vi "Pack5_UNDT.vi"(0 "data in":string="V4\u0012xV4\u0012\u0002\u0000\u0000\u0000pМC\u0016њwѕa\u0000\u0010\u0000‹\u0000\u0000\u0000\u0000\u0000\u0000\u0000\u0000\u0000\u0000\u0000\u0000\u0000\u0000\u0000\u0000\u0000\u0000\u0000\u0000o\u0012ѓ9\u0000\u0000\u0000\u0000\u0000\u0001\u0000\u0001+\u0019\u0000\u0001яя\"\"яяяяяяяяяяяяяяяяяяяяяяяяяяяяяяяяяяяяяяяяяяяяяяяяяяяяяяяяяяяяxV4\u0012\u0001\u0000\u0000\u0000pМC\u0016њwѕa\u0000\u0010\u0000‹\u0000\u0000\u0000\u0000\u0000\u0000\u0000\u0000\u0000\u0000\u0000\u0000\u0000\u0000\u0000\u0000\u0000\u0000\u0000\u0000o\u0012ѓ9\u0000\u0000\u0000\u0000\u0000\u0001\u0000\u0001+\u0019\u0000\u0001яя\"\u0011яяяяяяяяяяяяяяяяяяяяяяяяяяяяяяяяяяяяяяяяяяяяяяяяяяяяяяяяяяя", 5 "N tick":u8 format="%02x", 9 "OptionPACK5":T4={"MagicWordStr"="xV4\u0012", "Header size"=56, "Проверка CRC8"=TRUE, "Проверка конца пакета"=TRUE, "GainCompens"=FALSE, "Неотбрасывать BadEnd пакеты"=FALSE, "Неотбрасывать BadCRC пакеты"=FALSE, "Привести к 1"=FALSE, "GainCoef"=FALSE, "K_scale"=1.0, "ScaleOrdinate"=enum."Проценты"}, 11 "error in":errorcluster) -> (4 "data out":string, 6 "output cluster 2":T2 {"UNDT_Cluster"."Gain Coeff" format="%#_6e"; "UNDT_Cluster"."Reserve 1" format="%02x"; "UNDT_Cluster"."Mux TX/RX" format="%02x"; "UNDT_Cluster"."ScanDelay" format="%02x"; "UNDT_Cluster"."SamplingInterval" format="%#_6e"; "UNDT_Cluster"."Lose Packet" format="%08x"; "UNDT_Cluster"."EncodersParam2" format="%016x"; "UNDT_Cluster"."EncodersParam1" format="%016x"; "UNDT_Cluster"."CRC 8" format="%02x"; "UNDT_Cluster"."N chanel" format="%02x"; "UNDT_Cluster"."N tick" format="%02x"; "UNDT_Cluster"."Ncycle" format="%04x"; "UNDT_Cluster"."FrameFormatVersion" format="%02x"; "UNDT_Cluster"."MagicWord" format="%.0x"}, 8 "Status":T1={"CRC8Good"=TRUE, "PackEndGood"=TRUE, "MWFind"=TRUE, "PackToSmall"=FALSE, "offset"=4}, 10 "PackToSmall":bool, 15 "error out":errorcluster)   [LabVIEW 2017]
uses:
  Control_EU/OptionPACK5.ctl
  Control_EU/DataCluster.ctl
  Control_EU/UNDT_ClusterPackRevers (Type).ctl
  Control_EU/Status_pack5.ctl
panel:
  out "offset":i32=4
  out "SizeToSmall":bool
  out "OfsetEndPack":u32
  out "MWFind":bool=TRUE
  out "PackEndGood":bool=TRUE
  out "CRC8Good":bool=TRUE
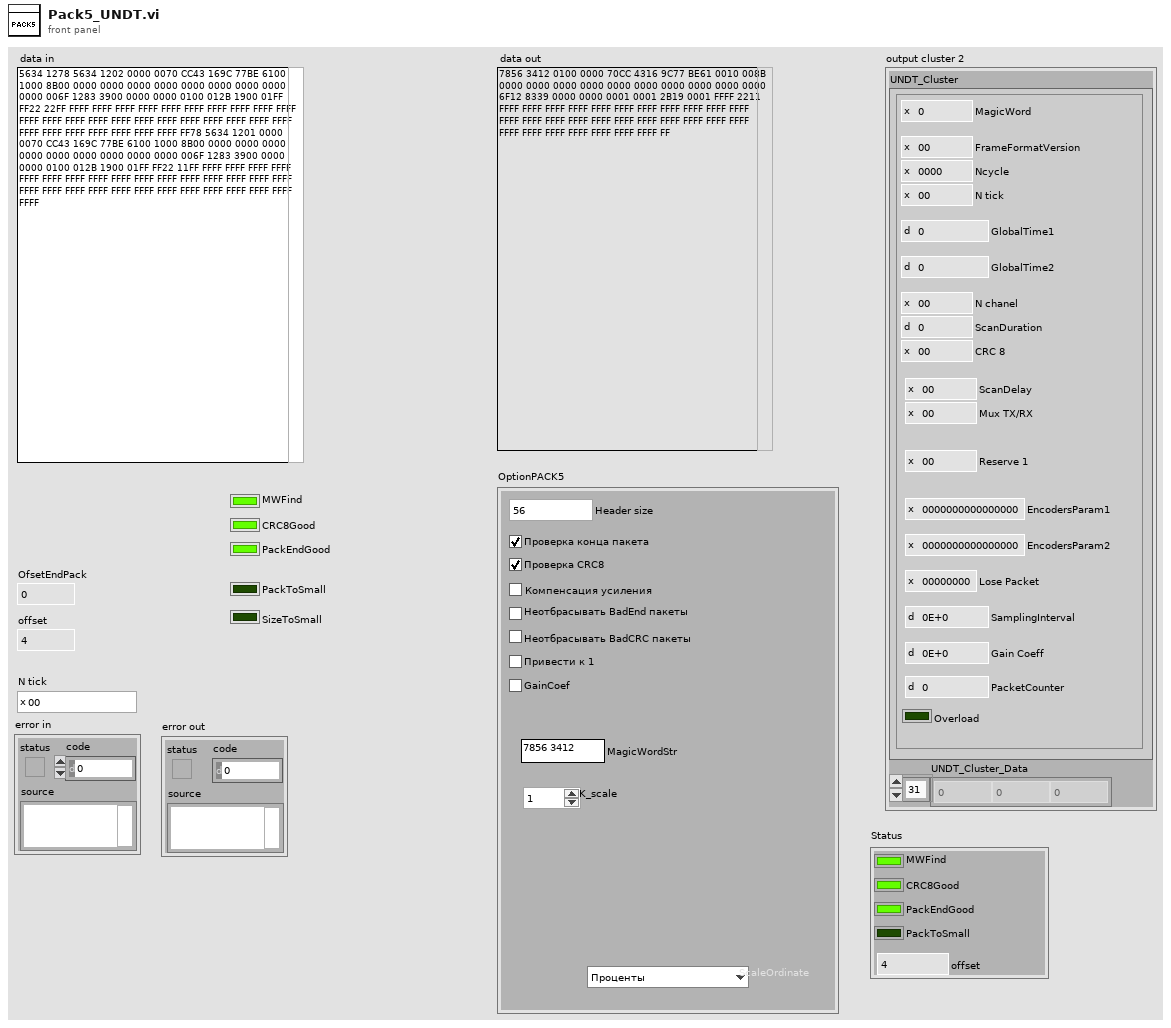
[diagram p1: front panel]
types:
  T1 = typedef "Status_pack5.ctl" = cluster{"CRC8Good":bool, "PackEndGood":bool, "MWFind":bool, "PackToSmall":bool, "offset":i32}
  T2 = typedef "DataCluster.ctl" = cluster{"UNDT_Cluster":T3, "UNDT_Cluster_Data":dbl[]}
  T3 = typedef "UNDT_ClusterPackRevers (Type).ctl" = cluster{"PacketCounter":u32, "Gain Coeff":sgl, "SamplingInterval":sgl, "Lose Packet":u32, "EncodersParam2":u64, "EncodersParam1":u64, "Reserve 1":u8, "Mux TX/RX":u8, "ScanDelay":u16, "CRC 8":u8, "ScanDuration":u16, "N chanel":u8, "GlobalTime2":u32, "GlobalTime1":u32, "N tick":u8, "Ncycle":u16, "FrameFormatVersion":u8, "MagicWord":u32, "Overload":bool}
  T4 = typedef "OptionPACK5.ctl" = cluster{"MagicWordStr":string, "Header size":u32, "Проверка CRC8":bool, "Проверка конца пакета":bool, "GainCompens":bool, "Неотбрасывать BadEnd пакеты":bool, "Неотбрасывать BadCRC пакеты":bool, "Привести к 1":bool, "GainCoef":bool, "K_scale":dbl, "ScaleOrdinate":enum16{"Отсчеты АЦП (±32767)", "Проценты", "Вольты", "дБмкВ (отн. 1 мкВ)", "Отсчеты АЦП (±1)"}}
  T5 = cluster{"CRC8Good":bool, "PackEndGood":bool, "MWFind":bool, "PackToSmall":bool, "offset past match":i32}
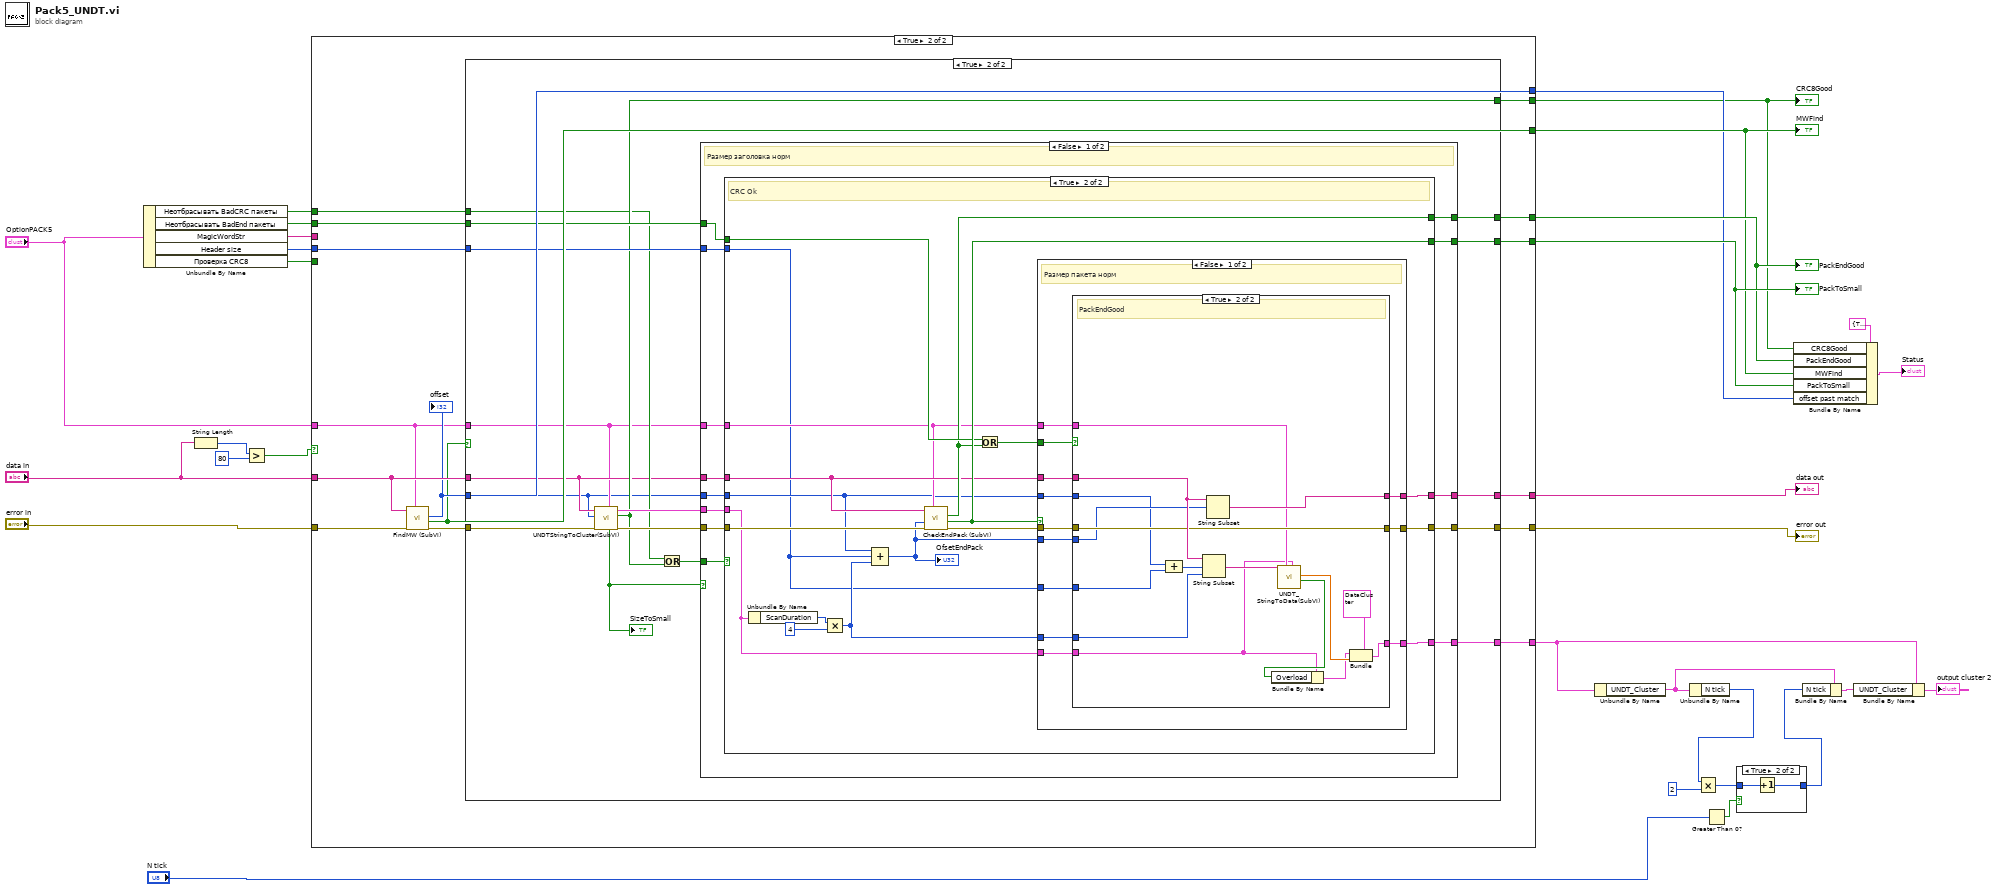
[diagram p0: block diagram]
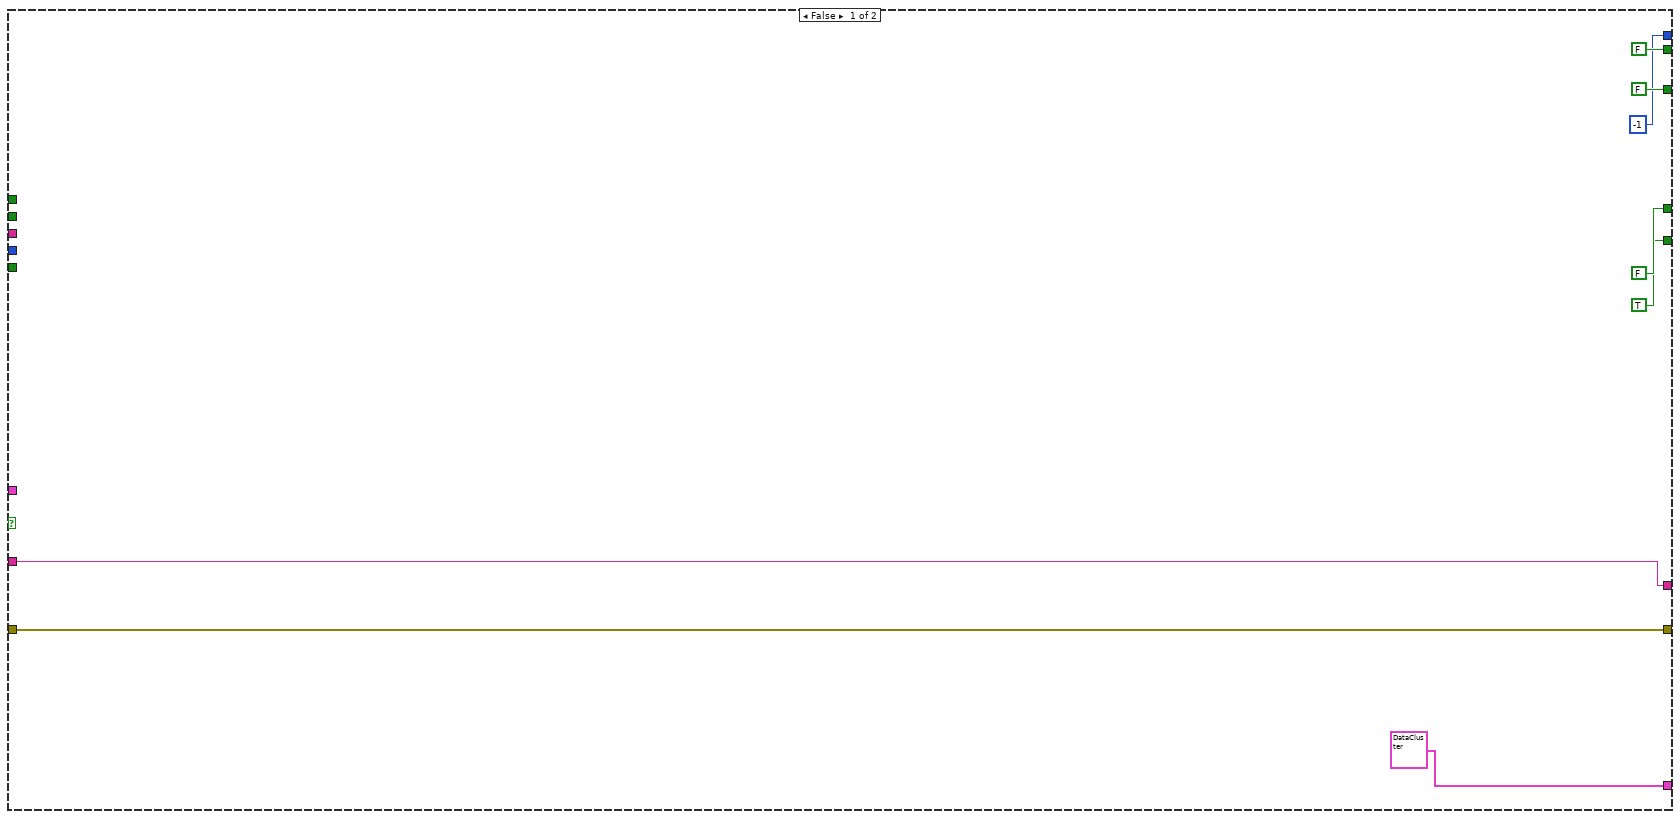
[diagram p3: hidden frame]
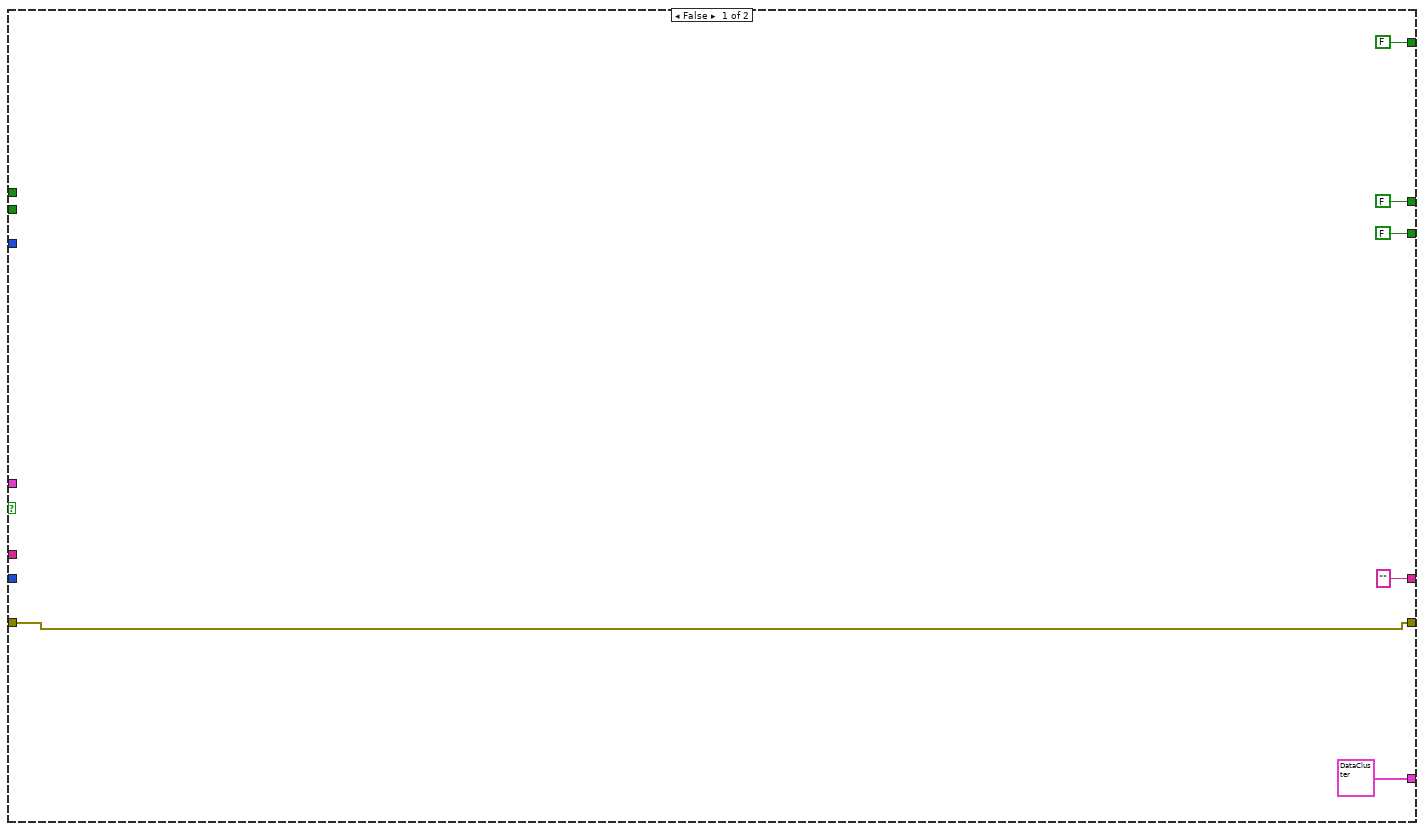
[diagram p4: hidden frame]
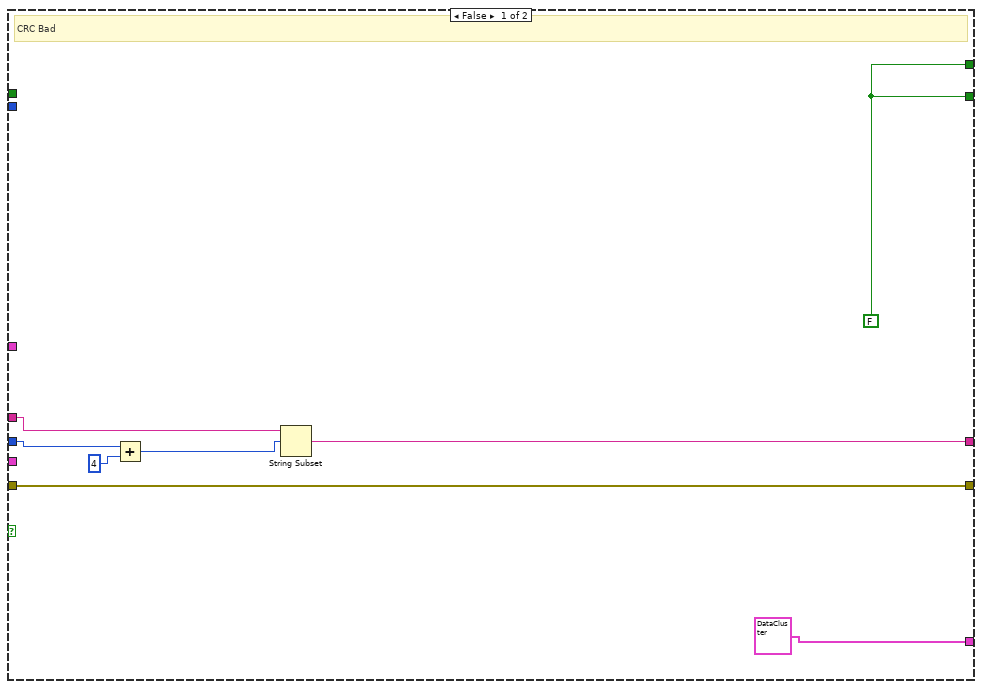
[diagram p5: hidden frame]
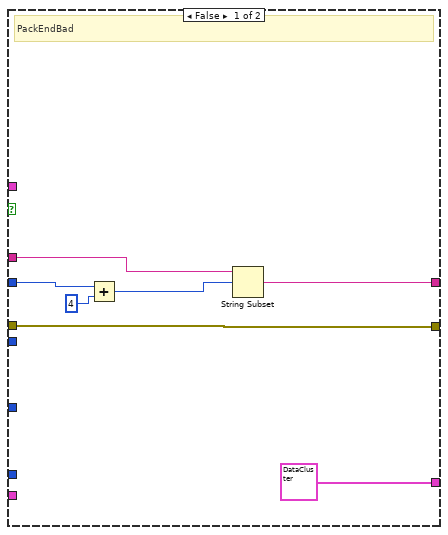
[diagram p6: hidden frame]
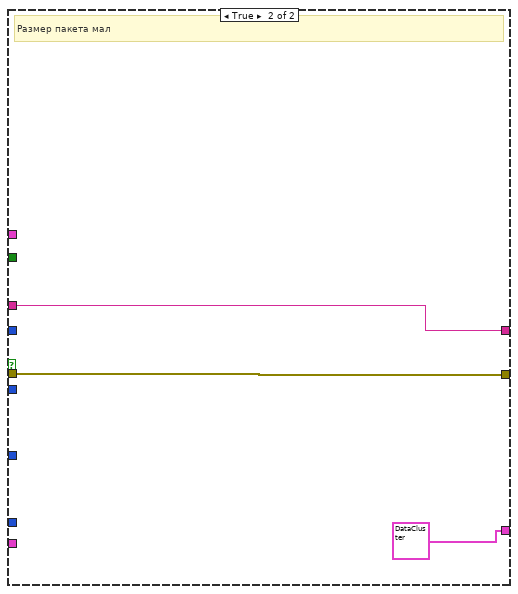
[diagram p7: hidden frame]
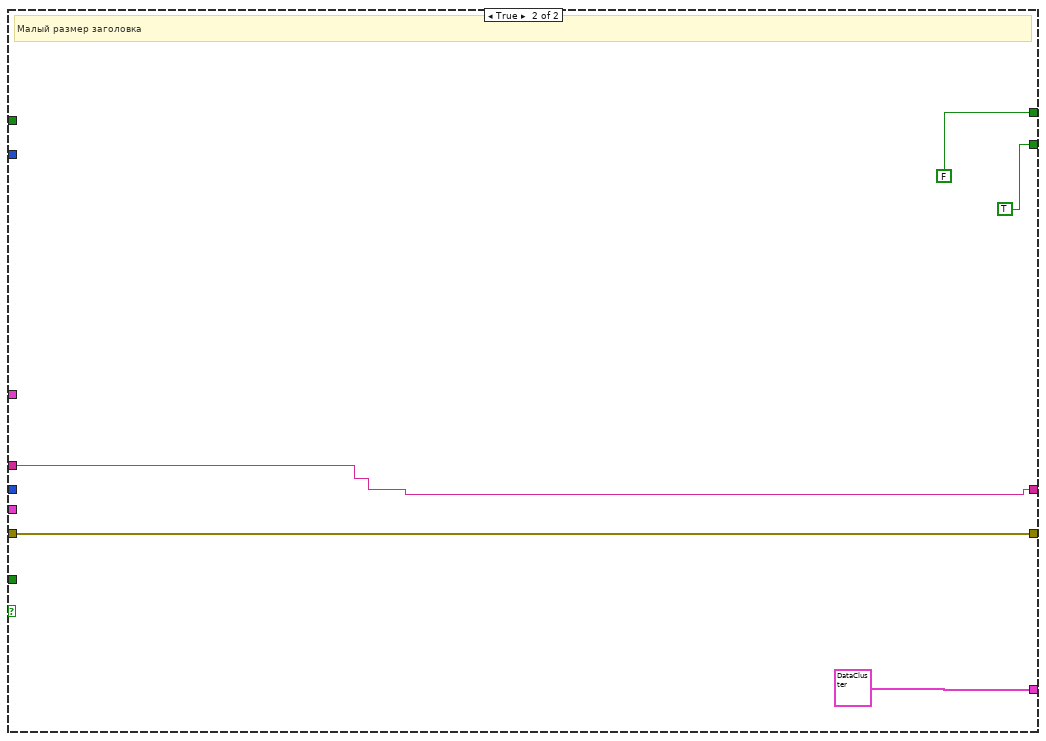
[diagram p8: hidden frame]
diagram:
  n1 = Unbundle By Name("OptionPACK5") -> ("Неотбрасывать BadCRC пакеты"=w12:bool, "Неотбрасывать BadEnd пакеты"=w14:bool, "MagicWordStr"=w27:string, "Header size"=w26:u32, "Проверка CRC8"=w25:bool)
  n2 = String Length(string="data in") -> (length=w10:i32)
  n3 = Greater?(x=w10, y=80) -> (0:w8:bool)
  n4 = case shown="True" w8 {
    tunnel: [w34 w42] -> w30
    tunnel: "error in" -> [w33 w52]
    tunnel: [w33 w51] -> w28
    tunnel: w27 -> [_ _]
    tunnel: w26 -> [_ w50]
    tunnel: w25 -> [_ _]
    tunnel: [T2 {"UNDT_Cluster"={"PacketCounter"=0, "Gain Coeff"=0.0, "SamplingInterval"=0.0, "Lose Packet"=0, "EncodersParam2"=0, "EncodersParam1"=0, "Reserve 1"=0, "Mux TX/RX"=0, "ScanDelay"=0, "CRC 8"=0, "ScanDuration"=0, "N chanel"=0, "GlobalTime2"=0, "GlobalTime1"=0, "N tick"=0, "Ncycle"=0, "FrameFormatVersion"=0, "MagicWord"=0, "Overload"=FALSE}, "UNDT_Cluster_Data"=[]} ("output cluster 2") w49] -> w24
    tunnel: [TRUE ("PackToSmall") w48] -> w18
    tunnel: [FALSE ("PackEndGood") w47] -> w17
    tunnel: [FALSE ("MWFind") w39] -> w16
    tunnel: [-1 ("offset past match") w41] -> w15
    tunnel: w14 -> [_ w46]
    tunnel: [FALSE ("CRC8Good") w45] -> w13
    tunnel: w12 -> [_ w44]
    tunnel: "data in" -> [w34 w43]
    tunnel: "OptionPACK5" -> [_ w40]
    frame False {
    }
    frame True {
      n5 = call "FindMW (SubVI).vi"("OptionPACK5"=w40, "error in"=w52, "string in"=w43) -> ("error out"=w53:errorcluster, "MWFind"=w39:bool, "offset"=w41:i32)  [unwired: 6 in]
      "offset" <- w41
      n6 = case shown="True" w39 {
        tunnel: w53 -> [w58 w74]
        tunnel: [w58 w73] -> w51
        tunnel: w50 -> [_ w72]
        tunnel: [T2 {"UNDT_Cluster"={"PacketCounter"=0, "Gain Coeff"=0.0, "SamplingInterval"=0.0, "Lose Packet"=0, "EncodersParam2"=0, "EncodersParam1"=0, "Reserve 1"=0, "Mux TX/RX"=0, "ScanDelay"=0, "CRC 8"=0, "ScanDuration"=0, "N chanel"=0, "GlobalTime2"=0, "GlobalTime1"=0, "N tick"=0, "Ncycle"=0, "FrameFormatVersion"=0, "MagicWord"=0, "Overload"=FALSE}, "UNDT_Cluster_Data"=[]} ("output cluster 2") w70] -> w49
        tunnel: [FALSE ("PackToSmall") w69] -> w48
        tunnel: [FALSE ("PackEndGood") w68] -> w47
        tunnel: w46 -> [_ w67]
        tunnel: [FALSE ("CRC8Good") w66] -> w45
        tunnel: w44 -> [_ w64]
        tunnel: w43 -> [_ w63]
        tunnel: ["" ("data in") w62] -> w42
        tunnel: w41 -> [_ w60]
        tunnel: w40 -> [_ w61]
        frame False {
        }
        frame True {
          n7 = call "UNDTStringToCluster(SubVI).vi"("OptionPACK5"=w61, "error in"=w74, "offset"=w60, "data_in"=w63) -> ("error out"=w75:errorcluster, "CRC8Good"=w66:bool, "UNDT_Cluster 3"=w71:T3, "SizeToSmall"=w76:bool)  [unwired: 4 in]
          "SizeToSmall" <- w76
          n8 = Or(x=w64, y=w66) -> (x .or. y?=w65:bool)
          n9 = case shown="False" w76 {
            tunnel: w72 -> [w89 _]
            tunnel: w75 -> [w88 w158]
            tunnel: w71 -> [w87 _]
            tunnel: [w85 w158] -> w73
            tunnel: w65 -> [w86 _]
            tunnel: [w84 T2 {"UNDT_Cluster"={"PacketCounter"=0, "Gain Coeff"=0.0, "SamplingInterval"=0.0, "Lose Packet"=0, "EncodersParam2"=0, "EncodersParam1"=0, "Reserve 1"=0, "Mux TX/RX"=0, "ScanDelay"=0, "CRC 8"=0, "ScanDuration"=0, "N chanel"=0, "GlobalTime2"=0, "GlobalTime1"=0, "N tick"=0, "Ncycle"=0, "FrameFormatVersion"=0, "MagicWord"=0, "Overload"=FALSE}, "UNDT_Cluster_Data"=[]} ("output cluster 2")] -> w70
            tunnel: [w83 FALSE ("PackEndGood")] -> w68
            tunnel: [w82 TRUE ("PackToSmall")] -> w69
            tunnel: w67 -> [w81 _]
            tunnel: w63 -> [w80 w154]
            tunnel: [w79 w154] -> w62
            tunnel: w61 -> [w78 _]
            tunnel: w60 -> [w77 _]
            frame False {
              # "Размер заголовка норм"
              n10 = case shown="True" w86 {
                tunnel: w89 -> [_ w98]
                tunnel: w88 -> [w96 w115]
                tunnel: w87 -> [_ w106]
                tunnel: [w97 w113] -> w79
                tunnel: [w96 w112] -> w85
                tunnel: [T2 {"UNDT_Cluster"={"PacketCounter"=0, "Gain Coeff"=0.0, "SamplingInterval"=0.0, "Lose Packet"=0, "EncodersParam2"=0, "EncodersParam1"=0, "Reserve 1"=0, "Mux TX/RX"=0, "ScanDelay"=0, "CRC 8"=0, "ScanDuration"=0, "N chanel"=0, "GlobalTime2"=0, "GlobalTime1"=0, "N tick"=0, "Ncycle"=0, "FrameFormatVersion"=0, "MagicWord"=0, "Overload"=FALSE}, "UNDT_Cluster_Data"=[]} ("output cluster 2") w111] -> w84
                tunnel: [w95 w107] -> w83
                tunnel: [w95 w110] -> w82
                tunnel: w81 -> [_ w108]
                tunnel: w80 -> [w93 w105]
                tunnel: w78 -> [_ w102]
                tunnel: w77 -> [w92 w100]
                frame False {
                  w95 = FALSE ("PackEndGood")
                  # "CRC Bad"
                  n11 = Add(x=w92, y=4 ("offset (0)")) -> (x+y=w90:i32)
                  n12 = String Subset(string=w93, offset (0)=w90) -> (substring=w97:string)  [unwired: 1 in]
                }
                frame True {
                  # "CRC Ok"
                  n13 = Unbundle By Name(w106) -> ("ScanDuration"=w104:u16)
                  n14 = Multiply(x=w104, y=4) -> (x*y=w101:i32)
                  n15 = Compound Arithmetic op=ADD(w100, w98, w101) -> (w99:u32)
                  "OfsetEndPack" <- w99
                  n16 = call "CheckEndPack (SubVI).vi"("OptionPACK5"=w102, "error in"=w115, "OfsetEndPack"=w99, "data"=w105) -> ("error out"=w114:errorcluster, "PackToSmall"=w110:bool, "PackEndGood"=w107:bool)  [unwired: 5 in]
                  n17 = Or(x=w108, y=w107) -> (x .or. y?=w109:bool)
                  n18 = case shown="False" w110 {
                    tunnel: w101 -> [w127 _]
                    tunnel: w106 -> [w126 _]
                    tunnel: w105 -> [w125 w152]
                    tunnel: w114 -> [w124 w153]
                    tunnel: [w123 w152] -> w113
                    tunnel: [w122 w153] -> w112
                    tunnel: w109 -> [w121 _]
                    tunnel: [w120 T2 {"UNDT_Cluster"={"PacketCounter"=0, "Gain Coeff"=0.0, "SamplingInterval"=0.0, "Lose Packet"=0, "EncodersParam2"=0, "EncodersParam1"=0, "Reserve 1"=0, "Mux TX/RX"=0, "ScanDelay"=0, "CRC 8"=0, "ScanDuration"=0, "N chanel"=0, "GlobalTime2"=0, "GlobalTime1"=0, "N tick"=0, "Ncycle"=0, "FrameFormatVersion"=0, "MagicWord"=0, "Overload"=FALSE}, "UNDT_Cluster_Data"=[]} ("output cluster 2")] -> w111
                    tunnel: w99 -> [w119 _]
                    tunnel: w102 -> [w118 _]
                    tunnel: w100 -> [w117 _]
                    tunnel: w98 -> [w116 _]
                    frame False {
                      # "Размер пакета норм"
                      n19 = case shown="True" w121 {
                        tunnel: w127 -> [_ w140]
                        tunnel: w126 -> [_ w135]
                        tunnel: w125 -> [w134 w150]
                        tunnel: w124 -> [w132 w142]
                        tunnel: [w133 w149] -> w123
                        tunnel: [w132 w142] -> w122
                        tunnel: [T2 {"UNDT_Cluster"={"PacketCounter"=0, "Gain Coeff"=0.0, "SamplingInterval"=0.0, "Lose Packet"=0, "EncodersParam2"=0, "EncodersParam1"=0, "Reserve 1"=0, "Mux TX/RX"=0, "ScanDelay"=0, "CRC 8"=0, "ScanDuration"=0, "N chanel"=0, "GlobalTime2"=0, "GlobalTime1"=0, "N tick"=0, "Ncycle"=0, "FrameFormatVersion"=0, "MagicWord"=0, "Overload"=FALSE}, "UNDT_Cluster_Data"=[]} ("output cluster 2") w147] -> w120
                        tunnel: w119 -> [_ w141]
                        tunnel: w118 -> [_ w139]
                        tunnel: w117 -> [w130 w138]
                        tunnel: w116 -> [_ w137]
                        frame False {
                          # "PackEndBad"
                          n20 = Add(x=w130, y=4 ("offset (0)")) -> (x+y=w128:i32)
                          n21 = String Subset(string=w134, offset (0)=w128) -> (substring=w133:string)  [unwired: 1 in]
                        }
                        frame True {
                          # "PackEndGood"
                          n22 = Compound Arithmetic op=ADD(w138, w137) -> (w136:u32)
                          n23 = String Subset(string=w150, offset (0)=w136, length (rest)=w140) -> (substring=w146:string)
                          n24 = String Subset(string=w150, offset (0)=w141) -> (substring=w149:string)  [unwired: 1 in]
                          n25 = call "UNDT_StringToData(SubVI).vi"("UNDT_Cluster 3"=w135, "OptionPACK5"=w139, "string in"=w146) -> ("Over"=w144:bool, "DataOut"=w148:dbl[])  [unwired: 7 in]
                          n26 = Bundle By Name(cluster=w135, "Overload"=w144) -> (w145:T3)
                          n27 = Bundle(cluster=T2 {"UNDT_Cluster"={"PacketCounter"=0, "Gain Coeff"=0.0, "SamplingInterval"=0.0, "Lose Packet"=0, "EncodersParam2"=0, "EncodersParam1"=0, "Reserve 1"=0, "Mux TX/RX"=0, "ScanDelay"=0, "CRC 8"=0, "ScanDuration"=0, "N chanel"=0, "GlobalTime2"=0, "GlobalTime1"=0, "N tick"=0, "Ncycle"=0, "FrameFormatVersion"=0, "MagicWord"=0, "Overload"=FALSE}, "UNDT_Cluster_Data"=[]} ("output cluster 2"), "UNDT_Cluster"=w145, "UNDT_Cluster_Data"=w148) -> (w147:T2)
                        }
                      }
                    }
                    frame True {
                      # "Размер пакета мал"
                    }
                  }
                }
              }
            }
            frame True {
              # "Малый размер заголовка"
            }
          }
        }
      }
    }
  }
  "CRC8Good" <- w13
  "data out" <- w30
  "error out" <- w28
  "MWFind" <- w16
  "PackEndGood" <- w17
  "PackToSmall" <- w18
  n28 = Unbundle By Name(w24) -> ("UNDT_Cluster"=w23:T3)
  n29 = Unbundle By Name(w23) -> ("N tick"=w4:u8)
  n30 = Multiply(x=w4, y=u8 2) -> (x*y=w5:u8)
  n31 = Greater Than 0?(x="N tick") -> (x > 0?=w1:bool)
  n32 = case shown="True" w1 {
    tunnel: w5 -> [w159 w161]
    tunnel: [w159 w160] -> w3
    frame False {
    }
    frame True {
      n33 = Increment(x=w161) -> (x+1=w160:u8)
    }
  }
  n34 = Bundle By Name(cluster=T5 {"CRC8Good"=TRUE, "PackEndGood"=TRUE, "MWFind"=TRUE, "PackToSmall"=FALSE, "offset past match"=0} ("Status"), "CRC8Good"=w13, "PackEndGood"=w17, "MWFind"=w16, "PackToSmall"=w18, "offset past match"=w15) -> (→"Status":T5)
  n35 = Bundle By Name(cluster=w23, "N tick"=w3) -> (w22:T3)
  n36 = Bundle By Name(cluster=w24, "UNDT_Cluster"=w22) -> (→"output cluster 2":T2)
